vi "OK.vi"(8 "error in (no error)":errorcluster, 11 "TouchScreen in":refnum<class "TouchScreen.lvclass">) -> (0 "error out":errorcluster, 3 "TouchScreen out":refnum<class "TouchScreen.lvclass">)   [LabVIEW 2020, in "TouchScreen.lvlib" / "TouchScreen.lvclass"]
uses:
  TouchScreen.lvclass
  C:/Program Files (x86)/National Instruments/LabVIEW 2020/vi.lib/ActorFramework/Actor/Actor.lvclass
  <vilib>/ActorFramework/Actor/Actor.lvclass/Actor.ctl
  TouchScreen.lvclass/TouchScreen.ctl
  TouchScreen Messages/new data number Msg/new data number Msg.lvclass/new data number Msg.ctl
  <vilib>/ActorFramework/Message Enqueuer/Message Enqueuer.lvclass/Message Enqueuer.ctl
  <vilib>/ActorFramework/Message Enqueuer/Enqueue.vi
  TouchScreen Messages/new data number Msg/new data number Msg.lvclass
  C:/Program Files (x86)/National Instruments/LabVIEW 2020/vi.lib/ActorFramework/Message/Message.lvclass
  <vilib>/ActorFramework/Message Priority Queue/Priority Enqueue.vi
  <vilib>/ActorFramework/Actor/Actor.lvclass
panel:
  out "number":string
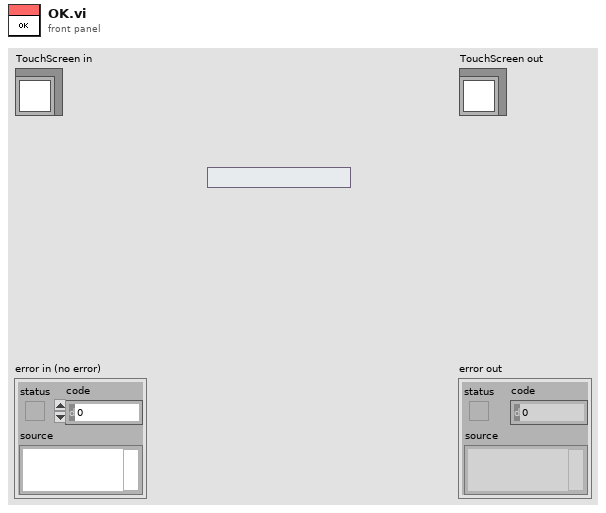
[diagram p1: front panel]
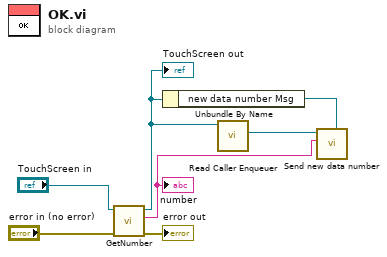
[diagram p0: block diagram]
diagram:
  n1 = call-dynamic "GetNumber.vi"("error in (no error)"="error in (no error)", "TouchScreen in"="TouchScreen in") -> ("error out"=→"error out":errorcluster, "number"=w3:string, "TouchScreen out"=w2:refnum<class "TouchScreen.lvclass">)  [unwired: 7 in]
  "TouchScreen out" <- w2
  "number" <- w3
  n2 = Unbundle By Name(w2) -> ("new data number Msg"=w1:refnum<class "new data number Msg.lvclass">)
  n3 = call <vilib>:"Read Caller Enqueuer.vi"("Actor"=w2) -> ("Caller Enqueuer"=w4:refnum<class "Message Enqueuer.lvclass">)  [unwired: 10 in]
  n4 = call "Send new data number.vi"("Message Type"=w1, "number"=w3, "Message Enqueuer"=w4) -> ()  [unwired: 7 in, 2 out]
